vi "Dependency Add RT Destination.vi"(7 "Supported Target Value":string, 8 "error in (no error)":errorcluster, 10 "Dependency ref in":refnum<k20>, 11 "XML File ref in":refnum<k20>) -> (0 "error out":errorcluster, 2 "Dependency ref out":refnum<k20>, 3 "XML File ref out":refnum<k20>)   [LabVIEW 2019, in "Project XML Editor.lvclass"]
uses:
  Project XML Editor.lvclass
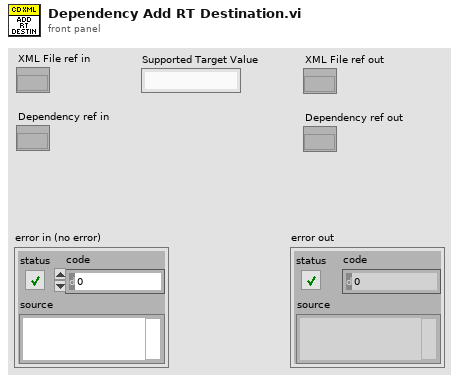
[diagram p1: front panel]
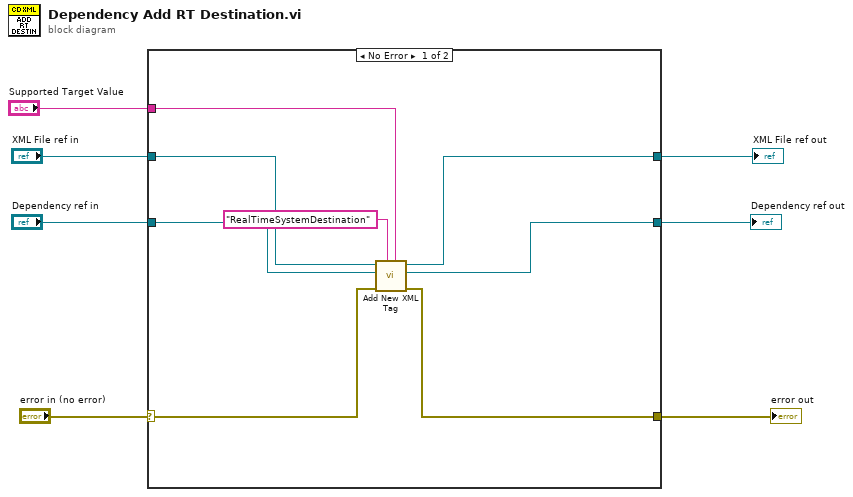
[diagram p0: block diagram]
diagram:
  n1 = case shown="No Error" "error in (no error)" {
    selector: "error in (no error)" -> [w8 w16]
    tunnel: "Supported Target Value" -> [w15 _]
    tunnel: "XML File ref in" -> [w13 w17]
    tunnel: "Dependency ref in" -> [w12 w18]
    tunnel: [w11 w18] -> w4
    tunnel: [w10 w17] -> w3
    tunnel: [w9 w16] -> w2
    frame No Error {
      n2 = call "Add New XML Tag.vi"("Tag Data"=w15, "Tag Name"="RealTimeSystemDestination", "error in (no error)"=w8, "Owning Element"=w12, "XML File Ref in"=w13) -> ("error out"=w9:errorcluster, "dup Owning Element"=w11:refnum<k20>, "XML File Ref out"=w10:refnum<k20>)  [unwired: 4 in]
    }
    frame Error {
    }
  }
  "Dependency ref out" <- w4
  "XML File ref out" <- w3
  "error out" <- w2
